vi "Find Workspace.vi"(8 "Error In":errorcluster, 10 "Control In":T2={"I-O.lvclass"=refnum, "Gantry"=refnum, "Dispenser"="COM1"}, 11 "Carrier Tray in":refnum<class "Assembly Tray.lvclass">) -> (0 "Error Out":errorcluster, 1 "Workspace":T1, 2 "Control Out":T2={"I-O.lvclass"=refnum, "Gantry"=refnum, "Dispenser"="COM1"}, 3 "Carrier Tray Out":refnum<class "Assembly Tray.lvclass">)   [LabVIEW 2020, in "Assembly Tray.lvclass"]
uses:
  Assembly Tray.lvclass
  Fixture.lvclass
  Controller/Controllers.ctl
  Controller/Controller.lvclass
  Workspace.ctl
  Controller/I-O/I-O.lvclass
  C:/Program Files (x86)/Aerotech/A3200/LabVIEW/2010/Bin/Aerotech.A3200.dll
  Program Files (x86)/Aerotech/A3200/LabVIEW/2010/Bin/Aerotech.A3200.dll
panel:
  out "XYZTheta Centers":dbl[][](array[numeric])
  in  "output cluster 2":T1
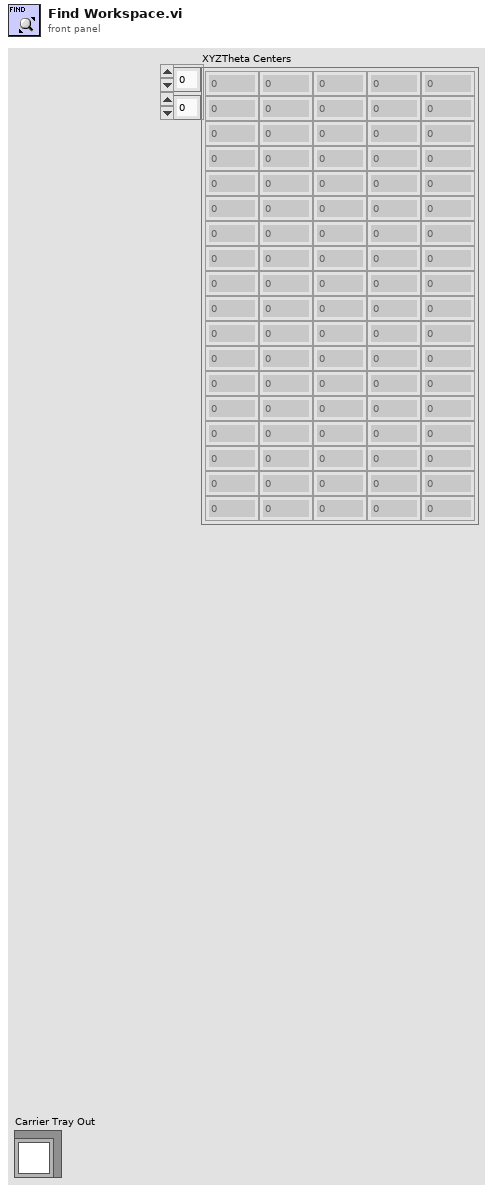
[diagram p1: front panel]
types:
  T1 = typedef "Fixture.lvclass/Workspace.ctl" = cluster{"XYZTheta":dbl[], "Workspace Valve":i32, "Workspace Sensor":i32}
  T2 = typedef "Controller.lvclass/Controllers.ctl" = cluster{"I-O.lvclass":refnum<class "I-O.lvclass">, "Gantry":refnum<k24>, "Dispenser":refnum<visa-resource-name>}
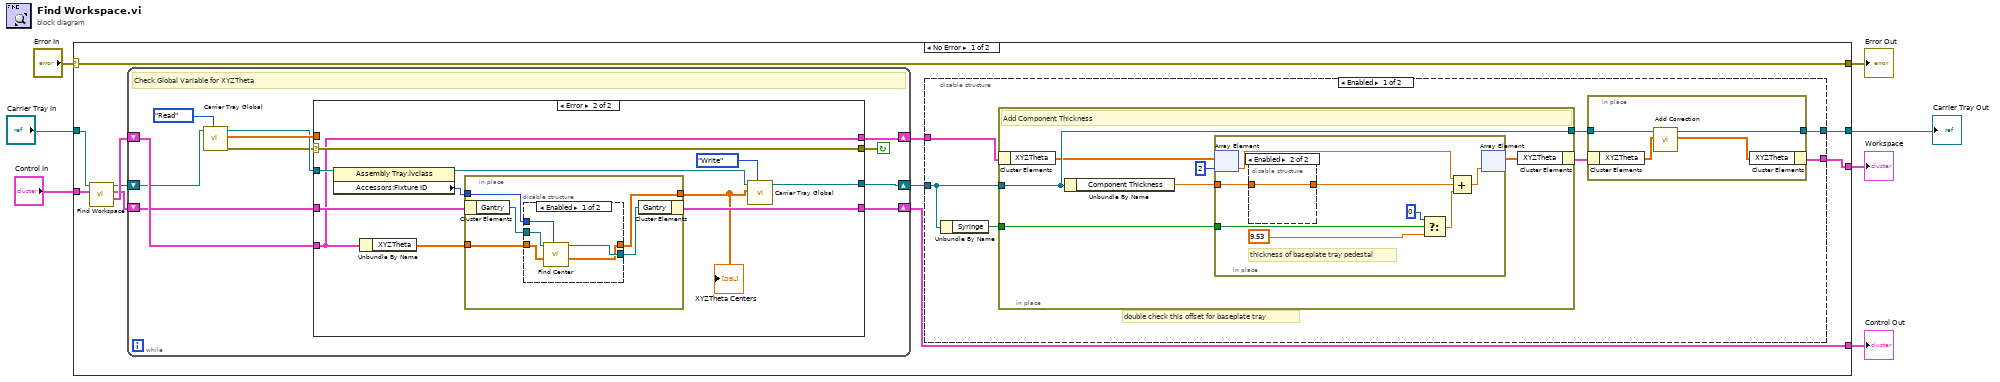
[diagram p0: block diagram]
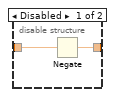
[diagram p2: hidden frame]
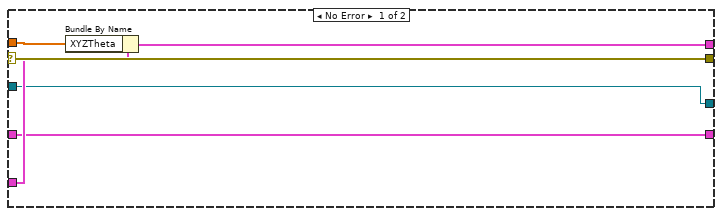
[diagram p4: hidden frame]
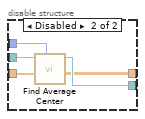
[diagram p5: hidden frame]
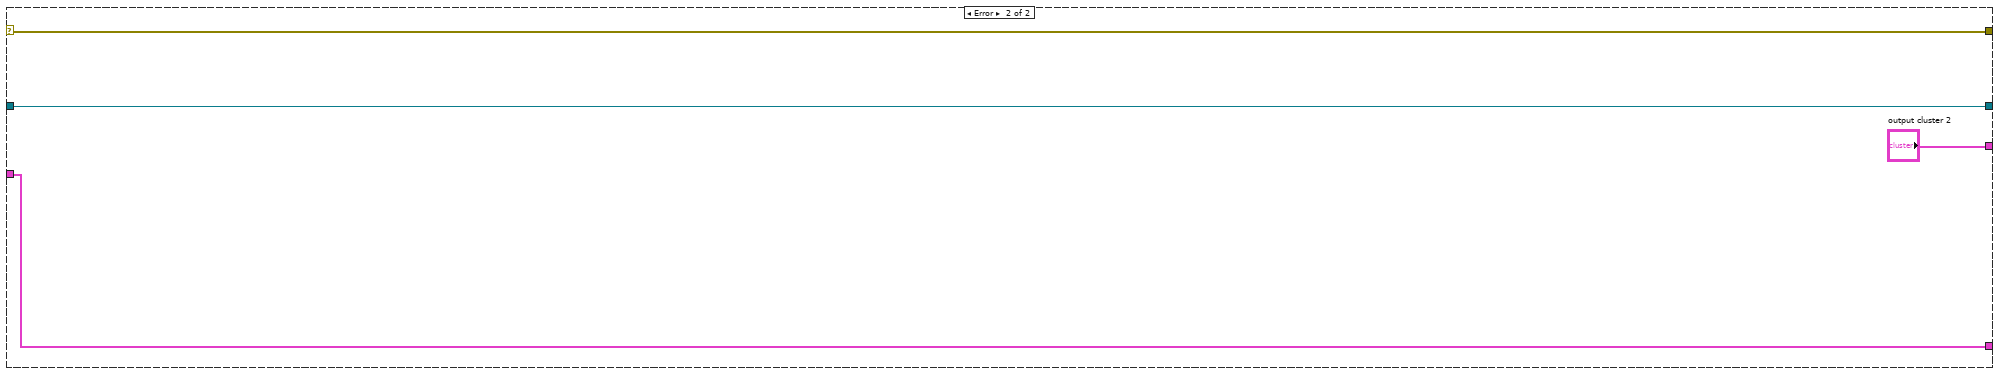
[diagram p6: hidden frame]
diagram:
  n1 = case shown="No Error" "Error In" {
    selector: "Error In" -> [w18 w94]
    tunnel: [w18 w94] -> w6
    tunnel: "Control In" -> [w17 w95]
    tunnel: [w13 w95] -> w4
    tunnel: "Carrier Tray in" -> [w16 w92]
    tunnel: [w14 "output cluster 2"] -> w2
    tunnel: [w15 w92] -> w1
    frame No Error {
      n2 = call-parent "Find Workspace.vi"("Control In"=w17, "Workspace In"=w16) -> (1:"Workspace Out"=w12:T1, "Control Out"=w11:T2, 3:"Workspace Out"=w8:refnum<class "Assembly Tray.lvclass">)  [unwired: 6 in, 1 out]
      n3 = while {
        shift-right: [w52] -> w10
        shift-left: w8 -> [w50]
        shift-right: [w54] -> w13
        shift-left: w11 -> [w55]
        shift-right: [w51] -> w9
        shift-left: w12 -> [w56]
        stop <- w58 continue-if-true
        # "Check Global Variable for XYZTheta"
        n4 = call "Carrier Tray Global.vi"("Action"=enum16{"Initialize", "Read", "Write"}."Read", "Carrier Tray.lvclass"=w50) -> ("error out"=w49:errorcluster, "XYZTheta out"=w57:dbl[], "Carrier Tray.lvclass 2"=w53:refnum<class "Assembly Tray.lvclass">)  [unwired: 7 in]
        n5 = case shown="Error" w49 {
          selector: w49 -> [w65 w76]
          tunnel: [w65 w76] -> w58
          tunnel: w57 -> [w64 _]
          tunnel: [w63 w66] -> w51
          tunnel: w56 -> [w62 w66]
          tunnel: w55 -> [w60 w70]
          tunnel: [w60 w69] -> w54
          tunnel: w53 -> [w61 w73]
          tunnel: [w61 w75] -> w52
          frame No Error {
            n6 = Bundle By Name(cluster=w62, "XYZTheta"=w64) -> (w63:T1)
          }
          frame Error {
            n7 = property class="Assembly Tray.lvclass"(reference=w73) -> (reference out=w72:refnum<class "Assembly Tray.lvclass">, "Accessors:Fixture ID"=w71:i32)  [unwired: 1 in, 1 out]
            n8 = Unbundle By Name(w66) -> ("XYZTheta"=w68:dbl[])
            n9 = in-place {
              in-place-border: w71 -> [w81]
              in-place-border: w68 -> [w78]
              in-place-border: [w77] -> w67
              n10 = in-place-cluster #1(w70) -> ("Gantry"=w80:refnum<k24>)
              n11 = disable-structure shown="Enabled" {
                disable-tunnel: w81 -> [w86 w87]
                disable-tunnel: w80 -> [w85 w91]
                disable-tunnel: [w84 w90] -> w79
                disable-tunnel: w78 -> [w83 w89]
                disable-tunnel: [w82 w88] -> w77
                frame Enabled {
                  n12 = call "Find Center.vi"("Tray Number"=w86, "XYZTheta"=w83, "Gantry In"=w85) -> ("XYZTheta Centers"=w82:dbl[][], "Gantry Out"=w84:refnum<k24>)  [unwired: 7 in]
                }
                frame Disabled {
                  n13 = call "Find Average Center.vi"("Tray Number"=w87, "XYZTheta"=w89, "Gantry In"=w91) -> ("XYZTheta Centers"=w88:dbl[][], "Gantry Out"=w90:refnum<k24>)  [unwired: 7 in]
                }
              }
              n14 = in-place-cluster #1("Gantry"=w79) -> (w69:T2)
            }
            "XYZTheta Centers" <- w67
            n15 = call "Carrier Tray Global.vi"("Action"=enum16{"Initialize", "Read", "Write"}."Write", "XYZTheta in"=w67, "Carrier Tray.lvclass"=w72) -> ("Carrier Tray.lvclass 2"=w75:refnum<class "Assembly Tray.lvclass">)  [unwired: 6 in, 2 out]
          }
        }
      }
      n16 = disable-structure shown="Enabled" {
        disable-tunnel: [w25 w47] -> w15
        disable-tunnel: [w24 w48] -> w14
        disable-tunnel: w10 -> [w23 w47]
        disable-tunnel: w9 -> [w22 w48]
        frame Enabled {
          # "double check this offset for baseplate tray"
          n17 = Unbundle By Name(w23) -> ("Syringe"=w21:bool)
          n18 = in-place {
            in-place-border: w23 -> [w32]
            in-place-border: [w32] -> w20
            in-place-border: w21 -> [w31]
            # "Add Component Thickness"
            n19 = in-place-cluster #2(w22) -> ("XYZTheta"=w30:dbl[])
            n20 = Unbundle By Name(w32) -> ("Component Thickness"=w33:dbl)
            n21 = in-place {
              in-place-border: w33 -> [w37]
              in-place-border: w31 -> [w42]
              # "thickness of baseplate tray pedestal"
              n22 = in-place-array #3(w30, 2) -> (w38:dbl)
              n23 = disable-structure shown="Enabled" {
                disable-tunnel: w37 -> [w45 w46]
                disable-tunnel: [w44 w46] -> w36
                frame Disabled {
                  n24 = Negate(x=w45) -> (-x=w44:dbl)
                }
                frame Enabled {
                }
              }
              n25 = Select(t=0, s=w42, f=9.53) -> (s? t:f=w39:dbl)
              n26 = Compound Arithmetic op=ADD(w38, w36, w39) -> (w43:dbl)
              n27 = in-place-array #3(w43) -> (w34:dbl[])  [unwired: 1 out]
            }
            n28 = in-place-cluster #2("XYZTheta"=w34) -> (w19:T1)
          }
          n29 = in-place {
            in-place-border: [w29] -> w25
            in-place-border: w20 -> [w28]
            n30 = in-place-cluster #4(w19) -> ("XYZTheta"=w27:dbl[])
            n31 = call "Add Correction.vi"("XYZTheta"=w27, "Carrier Tray in"=w28) -> ("XYZTheta Out"=w26:dbl[], "Carrier Tray out"=w29:refnum<class "Assembly Tray.lvclass">)  [unwired: 7 in, 1 out]
            n32 = in-place-cluster #4("XYZTheta"=w26) -> (w24:T1)
          }
        }
        frame Disabled {
        }
      }
    }
    frame Error {
    }
  }
  "Error Out" <- w6
  "Control Out" <- w4
  "Workspace" <- w2
  "Carrier Tray Out" <- w1
